vi "Gk_chain_L5_Z.vi"(4 "g(NMr)":dbl format="%#_13g") -> (1 "gk_chain":dbl[](array[numeric]))   [LabVIEW 2015]
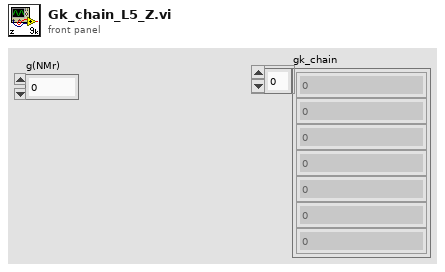
[diagram p1: front panel]
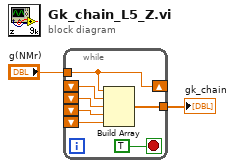
[diagram p0: block diagram]
diagram:
  n1 = while {
    tunnel: "g(NMr)" -> [w5]
    shift-right: [w5] -> _
    shift-left: _ -> [w9]
    shift-left: _ -> [w8]
    shift-left: _ -> [w7]
    shift-left: _ -> [w6]
    tunnel: [w4] -> w1
    stop <- TRUE stop-if-true
    n2 = Build Array(w5, w9, w8, w7, w6) -> (w4:dbl[])
  }
  "gk_chain" <- w1
